vi "End Bin.vi"   [LabVIEW 2018, in "Toolkit.lvlib" / "Reader.lvclass"]
doc: "Finishes reading a binary blob from the MessagePack data."
uses:
  Reader.lvclass
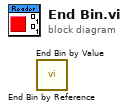
[diagram p0: block diagram]
diagram:
  n1 = call "End Bin by Reference.vi"() -> ()  [unwired: 10 in, 2 out]
  n2 = call "End Bin by Value.vi"() -> ()  [unwired: 10 in, 2 out]
